vi "ATEQwrite程序选择.vi"(6 "VISA resource name":refnum<visa-resource-name>="COM3" caption="COM", 7 "从站地址":u8=2 format="%x", 8 "baud rate (9600)":u32=9600 caption="波特率(9600)", 9 "The number of write":u16 format="%x", 10 "实际程序号-1":u16 format="%x", 11 "Write Address":u16 format="%x") -> (3 "Write Status":bool)   [LabVIEW 2014]
uses:
  <vilib>/Instr/_visa.llb/VISA Configure Serial Port (Instr).vi
panel:
  out "ReturnWrite":string
  out "WriteSend":string
  out "Write Return Value":string
  out "Send Write Date":string
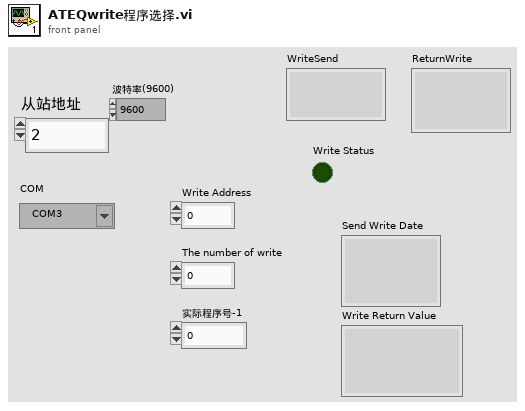
[diagram p1: front panel]
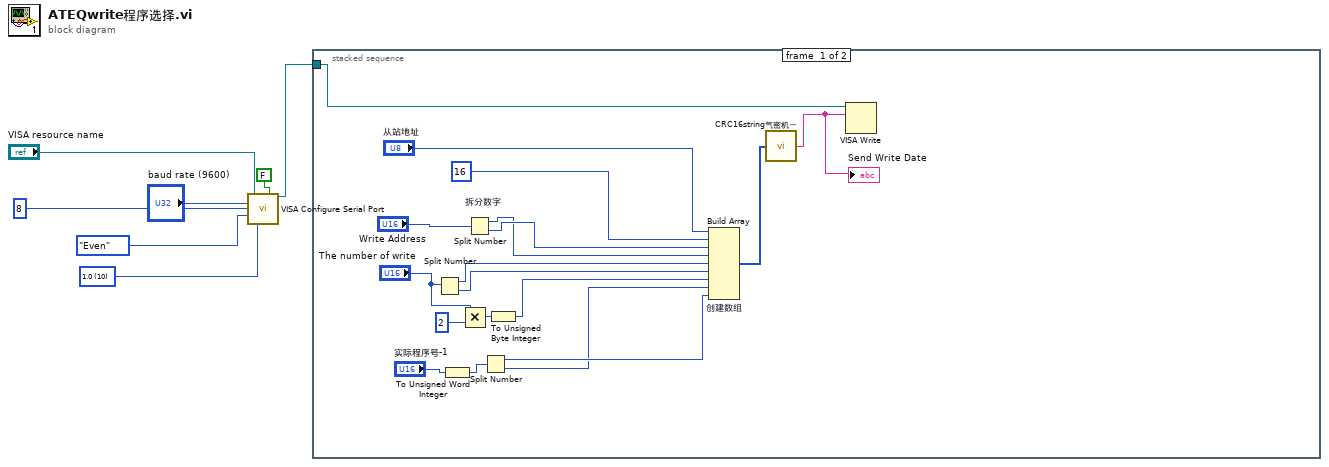
[diagram p0: block diagram]
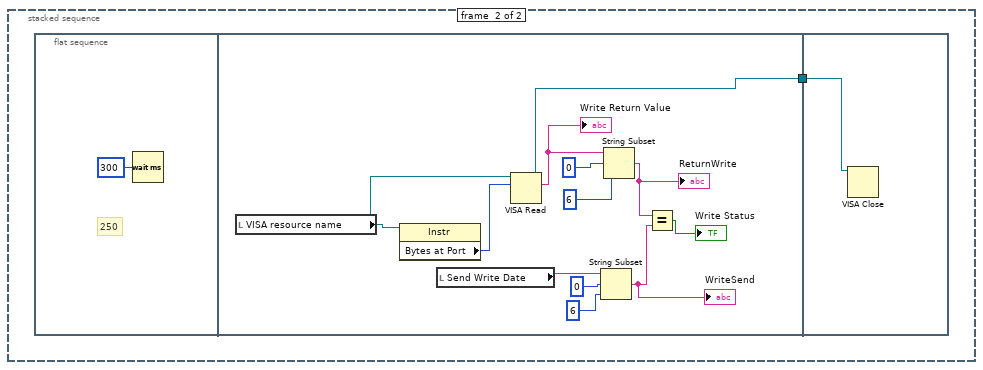
[diagram p2: hidden frame]
diagram:
  w7 = u16 10 items=["1.0"=10, "1.5"=15, "2.0"=20] ("stop bits (10: 1 bit)")
  n1 = call-poly "VISA Configure Serial Port"("VISA resource name"="VISA resource name", "Enable Termination\nChar (T)"=FALSE ("Enable Termination\nChar (T)"), "baud rate (9600)"="baud rate (9600)", "data bits (8)"=u16 8, "parity (0:none)"=enum16{"None", "Odd", "Even", "Mark", "Space"}."Even", "stop bits (10: 1 bit)"=w7) -> ("VISA resource name out"=w3:refnum<visa-resource-name>)  [unwired: 8 in, 1 out]
  n2 = stacked-sequence {
    tunnel: w3 -> [w22 _]
    frame #0 {
      n3 = Split Number(x="The number of write") -> (hi(x)=w21:u8, lo(x)=w20:u8)
      n4 = To Unsigned Word Integer(number="实际程序号-1") -> (unsigned 16bit integer=w25:u16)
      n5 = Multiply(x="The number of write", y=u16 2) -> (x*y=w16:u16)
      n6 = Split Number "拆分数字"(x="Write Address") -> (hi(x)=w9:u8, lo(x)=w10:u8)
      n7 = Split Number(x=w25) -> (hi(x)=w19:u8, lo(x)=w18:u8)
      n8 = To Unsigned Byte Integer(number=w16) -> (unsigned 8bit integer=w15:u8)
      n9 = Build Array "创建数组"("从站地址", u8 16, w10, w9, w21, w20, w15, w18, w19) -> (w23:u8[])
      n10 = call "CRC16string气密机一.vi"("数组"=w23) -> ("要发送的数据"=w11:string)
      "Send Write Date" <- w11
      n11 = VISA Write(VISA resource name=w22, write buffer=w11) -> ()  [unwired: 1 in, 3 out]
    }
    frame #1 {
      n12 = flat-sequence {
        tunnel: [w28] -> w26
        tunnel: w26 -> [w40]
        frame #0 {
          # "250"
          n13 = Wait (ms)(milliseconds to wait=u32 300 ("等待时间（毫秒）")) -> ()  [unwired: 1 out]
        }
        frame #1 {
          n14 = local read "VISA resource name"() -> (w39:refnum<visa-resource-name>)
          n15 = property class="Instr"(reference=w39) -> ("Bytes at Port"=w38:u32)  [unwired: 1 in, 2 out]
          n16 = local read "Send Write Date"() -> (w36:string)
          n17 = VISA Read(VISA resource name=w39, byte count=w38) -> (VISA resource name out=w28:refnum<visa-resource-name>, read buffer=w35:string)  [unwired: 1 in, 2 out]
          "Write Return Value" <- w35
          n18 = String Subset(string=w36, offset (0)=0 ("偏移量(0)"), length (rest)=6 ("长度（剩余）")) -> (substring=w31:string)
          "WriteSend" <- w31
          n19 = String Subset(string=w35, offset (0)=0 ("偏移量(0)"), length (rest)=6 ("长度（剩余）")) -> (substring=w32:string)
          "ReturnWrite" <- w32
          n20 = Equal?(x=w32, y=w31) -> (x = y?=→"Write Status":bool)
        }
        frame #2 {
          n21 = VISA Close(VISA resource name=w40) -> ()  [unwired: 1 in, 1 out]
        }
      }
    }
  }
